vi "Actor Core.vi"(8 "error in":errorcluster, 11 "Counter in":refnum<class "Counter.lvclass">) -> (0 "error out":errorcluster, 3 "Actor out":refnum<class "Actor.lvclass">)   [LabVIEW 2018, in "Feeder Actor.lvlib" / "Counter.lvclass"]
doc: "The user interface for this panel.\n\n----\nPlease see the following web address for additional documentation and tutorial information:\nhttp://www.mooregoodideas.com/mgi-panel-manager/\n\nAuthor: Derek Trepanier\n\nCopyright (c) 2018, Moore Good Ideas, Inc.\n\nAll rights reserved.\n\nRedistribution and use in source and binary forms, with or without modification, are permitted provided that the following conditions are met:\n\n * Redistributions of source code must retain the above copyright notice, this list of conditions and the following disclaimer.\n * Redistributions in binary form must reproduce the above copyright notice, this list of conditions and the following disclaimer in the documentation and/or other materials provided with the distribution.\n * Neither the name of Moore Good Ideas, Inc. nor the names of its contributors may be used to endorse or promote products derived from this software without specific prior written permission.\n\nTHIS SOFTWARE IS PROVIDED BY THE COPYRIGHT HOLDERS AND CONTRIBUTORS \"AS IS\" AND ANY EXPRESS OR IMPLIED WARRANTIES, INCLUDING, BUT NOT LIMITED TO, THE IMPLIED WARRANTIES OF MERCHANTABILITY AND FITNESS FOR A PARTICULAR PURPOSE ARE DISCLAIMED. IN NO EVENT SHALL THE COPYRIGHT OWNER OR CONTRIBUTORS BE LIABLE FOR ANY DIRECT, INDIRECT, INCIDENTAL, SPECIAL, EXEMPLARY, OR CONSEQUENTIAL DAMAGES (INCLUDING, BUT NOT LIMITED TO, PROCUREMENT OF SUBSTITUTE GOODS OR SERVICES; LOSS OF USE, DATA, OR PROFITS; OR BUSINESS INTERRUPTION) HOWEVER CAUSED AND ON ANY THEORY OF LIABILITY, WHETHER IN CONTRACT, STRICT LIABILITY, OR TORT (INCLUDING NEGLIGENCE OR OTHERWISE) ARISING IN ANY WAY OUT OF THE USE OF THIS SOFTWARE, EVEN IF ADVISED OF THE POSSIBILITY OF SUCH DAMAGE."
uses:
  Counter.lvclass
  C:/Program Files/National Instruments/LabVIEW 2018/vi.lib/MGI/Panel Manager/Panel Actor/Panel Actor/Panel Actor.lvclass
  <vilib>/ActorFramework/Actor/Actor.lvclass
  Counter.lvclass/Counter.ctl
  <vilib>/ActorFramework/Message Enqueuer/Message Enqueuer.lvclass/Message Enqueuer.ctl
  <vilib>/ActorFramework/Message Enqueuer/Enqueue.vi
  <vilib>/ActorFramework/Stop Msg/Stop Msg.lvclass
  C:/Program Files/National Instruments/LabVIEW 2018/vi.lib/ActorFramework/Message/Message.lvclass
  <vilib>/ActorFramework/Message Priority Queue/Priority Enqueue.vi
  <vilib>/MGI/Panel Manager/Panel Actor/Panel Actor/Panel Actor.lvclass
  Counter Messages/Set Counter Msg/Set Counter Msg.lvclass
  ADM/Main.lvlib
panel:
  in  "Counter":dbl(knob) caption="Mixer" scale=0.075..0.095
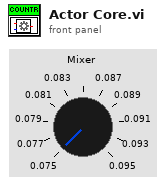
[diagram p1: front panel]
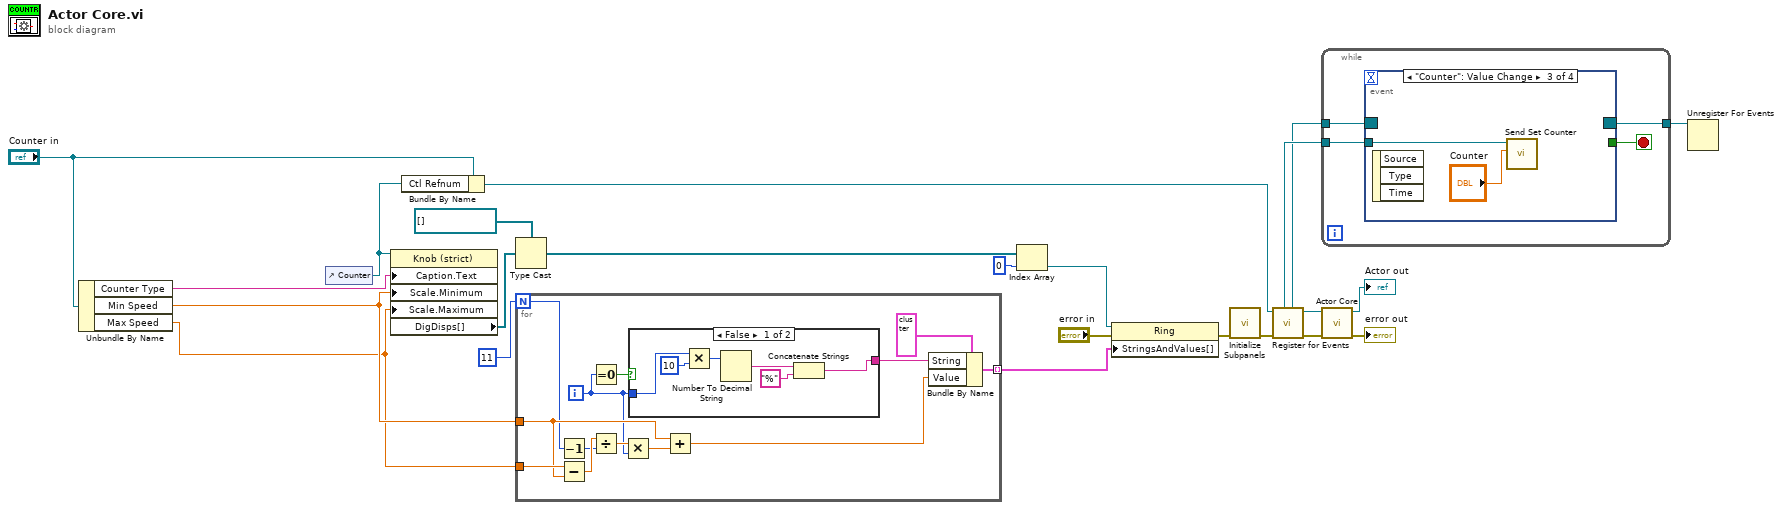
[diagram p0: block diagram]
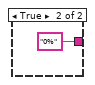
[diagram p2: hidden frame]
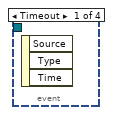
[diagram p3: hidden frame]
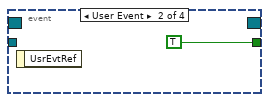
[diagram p4: hidden frame]
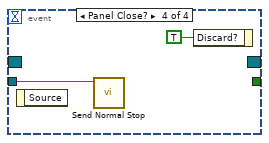
[diagram p5: hidden frame]
diagram:
  n1 = Unbundle By Name("Counter in") -> ("Counter Type"=w5:string, "Min Speed"=w2:dbl, "Max Speed"=w1:dbl)
  n2 = control-ref of="Counter"() -> (w6:refnum<vi>)
  n3 = property on="Property Node" class="Knob (strict)"(reference=w6, "Caption.Text"=w5, "Scale.Minimum"=w2, "Scale.Maximum"=w1) -> ("DigDisps[]"=w13:refnum<vi>[])  [unwired: 1 in, 2 out]
  n4 = Bundle By Name(cluster="Counter in", "Ctl Refnum"=w6) -> (w16:refnum<class "Counter.lvclass">)
  n5 = Type Cast(type=refnum<vi>[] [] ("Array"), x=w13) -> (*(type *) &x=w11:refnum<vi>[])
  n6 = for {
    N: 11 -> [w31]
    tunnel: [w35] -> w7 mode=indexing
    tunnel: w2 -> [w33]
    tunnel: w1 -> [w34]
    i -> [w24]
    n7 = Decrement(x=w31) -> (x-1=w30:i32)
    n8 = Subtract(x=w34, y=w33) -> (x-y=w32:dbl)
    n9 = Equal To 0?(x=w24) -> (x = 0?=w26:bool)
    n10 = Divide(x=w32, y=w30) -> (x/y=w29:dbl)
    n11 = Multiply(x=w29, y=w24) -> (x*y=w28:dbl)
    n12 = case shown="False" w26 {
      tunnel: [w37 "0%"] -> w25
      tunnel: w24 -> [w42 _]
      frame False {
        n13 = Multiply(x=w42, y=10) -> (x*y=w40:i32)
        n14 = Number To Decimal String(number=w40) -> (decimal integer string=w39:string)  [unwired: 1 in]
        n15 = Concatenate Strings(w39, "%" ("string")) -> (w37:string)
      }
      frame True {
      }
    }
    n16 = Add(x=w33, y=w28) -> (x+y=w27:dbl)
    n17 = Bundle By Name(cluster=cluster{"String":string, "Value":ext} {"String"="", "Value"=0.0} ("Cluster"), "String"=w25, "Value"=w27) -> (w35:cluster{"String":string, "Value":ext})
  }
  n18 = Index Array(array=w11, index=0) -> (element=w9:refnum<vi>)
  n19 = property class="Ring"(reference=w9, error in="error in", "StringsAndValues[]"=w7) -> (error out=w4:errorcluster)  [unwired: 1 out]
  n20 = call "Initialize Subpanels.vi"("error in (no error)"=w4) -> ("error out"=w14:errorcluster)  [unwired: 10 in]
  n21 = call <vilib>:"Register for Events.vi"("Error In"=w14, "Panel Actor in"=w16) -> ("Error Out"=w17:errorcluster, "Panel Actor out"=w18:refnum<class "Counter.lvclass">, "Pnl Actor"=w19:refnum<event-registration>, "Self Enqueuer"=w20:refnum<class "Message Enqueuer.lvclass">)  [unwired: 6 in]
  n22 = while {
    tunnel: w19 -> [w47]
    tunnel: w20 -> [w46]
    tunnel: [w44] -> w21
    stop <- w45 stop-if-true
    n23 = event shown="[2] \"Counter\": Value Change" {
      selector: w47 -> [_ _ _ _]
      dyn-events: [_ _ _ _] -> w44
      timeout: _ -> [_ _ _ _]
      tunnel: w46 -> [_ _ w49 w52]
      tunnel: [_ TRUE _ _] -> w45
      event Timeout {
        n24 = event-data() -> ()  [unwired: 1 in, 3 out]
      }
      event User Event {
        n25 = event-data() -> ()  [unwired: 1 in, 1 out]
      }
      event "Counter": Value Change {
        n26 = event-data() -> ()  [unwired: 1 in, 3 out]
        n27 = call "Send Set Counter.vi"("Input"="Counter", "Message Enqueuer in"=w49) -> ()  [unwired: 8 in, 2 out]
      }
      event Panel Close? {
        n28 = event-data() -> ()  [unwired: 1 in, 1 out]
        n29 = call <vilib>:"Send Normal Stop.vi"("Message Enqueuer"=w52) -> ()  [unwired: 10 in, 1 out]
        n30 = event-data("Discard?"=TRUE) -> ()  [unwired: 1 in, 1 out]
      }
    }
  }
  n31 = call-parent "Actor Core.vi"("error in"=w17, "Panel Actor in"=w18) -> ("error out"=→"error out":errorcluster, "Actor out"=→"Actor out":refnum<class "Actor.lvclass">)  [unwired: 8 in]
  n32 = Unregister For Events(event registration refnum=w21) -> ()  [unwired: 1 in, 1 out]
